vi "OnValueChange_System.vi"(8 "error in (no error)":errorcluster, 9 "Value":bool, 10 "Engine":refnum<class "Engine.lvclass">, 11 "Game in":refnum<class "Game.lvclass">) -> (0 "error out":errorcluster, 2 "Engine out":refnum<class "Engine.lvclass">, 3 "Game out":refnum<class "Game.lvclass">)   [LabVIEW 2019, in "RT_Game.lvlib" / "Game.lvclass"]
uses:
  Game.lvclass
  Engine/Engine.lvclass
  Game.lvclass/Game.ctl
  Menu/States.ctl
  GameMenu/GameMenu.lvclass/GameMenu.ctl
  GameMenu/Read Active_.vi
  GameMenu/GameMenu.lvclass
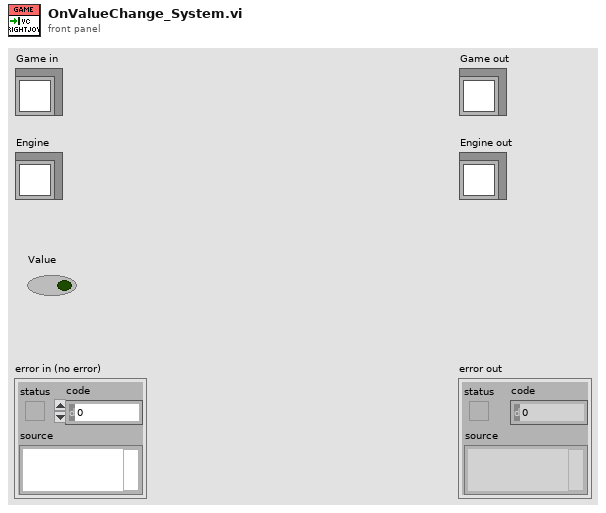
[diagram p1: front panel]
types:
  T1 = typedef "RT_Game.lvlib/Game.lvclass/States.ctl" = enum16{"Init", "Restart", "Menu", "Game", "Resume", "ToggleSingleplayer", "LoadNextGame", "ExitToMenu", "NewHighscore", "GameOver", "SlideOut"}
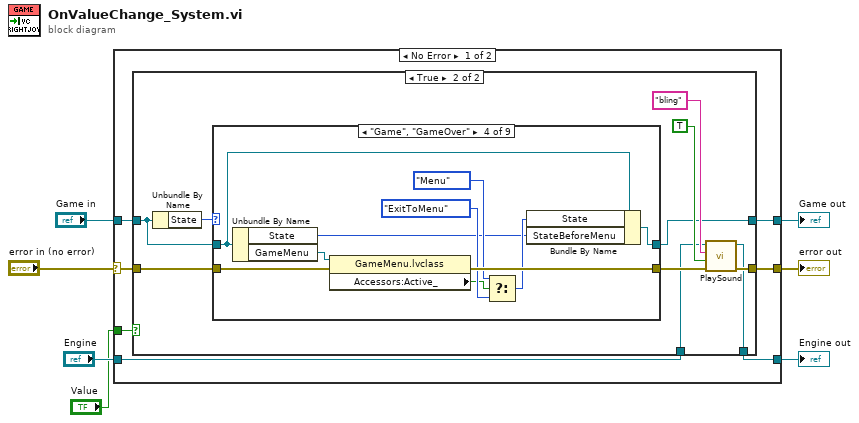
[diagram p0: block diagram]
diagram:
  n1 = case shown="No Error" "error in (no error)" {
    selector: "error in (no error)" -> [w12 w56]
    tunnel: [w13 w56] -> w6
    tunnel: [w14 w55] -> w4
    tunnel: "Game in" -> [w11 w55]
    tunnel: "Engine" -> [w8 w54]
    tunnel: [w9 w54] -> w2
    tunnel: "Value" -> [w10 _]
    frame No Error {
      n2 = case shown="True" w10 {
        tunnel: [w17 w20] -> w14
        tunnel: [w16 w24] -> w13
        tunnel: w12 -> [w16 w23]
        tunnel: w11 -> [w17 w22]
        tunnel: w8 -> [w15 w19]
        tunnel: [w15 w18] -> w9
        frame False {
        }
        frame True {
          n3 = Unbundle By Name(w22) -> ("State"=w21:T1)
          n4 = case shown="\"Game\", \"GameOver\"" w21 {
            tunnel: [w28 w30 w32 w43 w44 w46 w48 w50 w52] -> w25
            tunnel: w23 -> [w28 w30 w32 w42 w44 w46 w48 w50 w52]
            tunnel: w22 -> [w29 w31 w33 w36 w45 w47 w49 w51 w53]
            tunnel: [w29 w31 w33 w35 w45 w47 w49 w51 w53] -> w20
            frame "Init", Default {
            }
            frame "Restart" {
            }
            frame "Menu" {
            }
            frame "Game", "GameOver" {
              n5 = Unbundle By Name(w36) -> ("State"=w34:T1, "GameMenu"=w37:refnum<class "GameMenu.lvclass">)
              n6 = property class="GameMenu.lvclass"(reference=w37, error in=w42) -> (error out=w43:errorcluster, "Accessors:Active_"=w40:bool)  [unwired: 1 out]
              n7 = Select(t=States."Menu" ("State"), s=w40, f=States."ExitToMenu") -> (s? t:f=w38:T1)
              n8 = Bundle By Name(cluster=w36, "State"=w38, "StateBeforeMenu"=w34) -> (w35:refnum<class "Game.lvclass">)
            }
            frame "Resume" {
            }
            frame "ToggleSingleplayer" {
            }
            frame "LoadNextGame" {
            }
            frame "ExitToMenu" {
            }
            frame "SlideOut" {
            }
          }
          n9 = call "PlaySound.vi"("error in (no error)"=w25, "Overwrite"=TRUE, "Name"="bling", "Engine in"=w19) -> ("error out"=w24:errorcluster, "Engine out"=w18:refnum<class "Engine.lvclass">)  [unwired: 6 in]
        }
      }
    }
    frame Error {
    }
  }
  "error out" <- w6
  "Game out" <- w4
  "Engine out" <- w2
